vi "Smarthome - server.vi"() -> ()   [LabVIEW 2013]
panel:
  out "URL":string="C:\\Users\\kiat\\Downloads\\asd.mp4"
  in  "WindowsMediaPlayer":refnum<k7>(container)
  out "temperature level 3":bool
  out "Numeric 3":i32
  in  "Slide 3":dbl(slide) scale=16.0..27.0
  out "Ring 6":u16(ring)
  out "check for level 3":bool
  in  "Slide 2":dbl(slide) scale=16.0..27.0
  out "temperature level 2":bool
  out "Numeric 2":i32
  out "Ring 5":u16(ring)
  out "check for level 2":bool
  out "check for level":bool
  in  "Slide":dbl(slide) scale=16.0..27.0
  out "Numeric":i32
  out "temperature level":bool
  out "Ring 4":u16(ring)
  out "Boolean 16":bool
  out "start time 2":string
  out "end time 2":string
  out "Boolean 17":bool
  out "start time 3":string
  out "end time 3":string
  out "end time":string
  out "start time":string
  out "indicator - hour":bool
  out "Bedroom 2":bool
  out "Bedroom 1":bool
  out "Masterroom":bool
  out "For loop count - hour":i32
  in  "stop 3":bool
  out "hour":i32
  out "Ring 3":u16(ring)
  out "Ring 2":u16(ring)
  out "Boolean 15":bool
  in  "stop 2":bool
  out "Boolean 14":bool
  out "Boolean 13":bool
  out "Boolean 12":bool
  out "Boolean 11":bool
  out "Boolean 10":bool
  out "Boolean 9":bool
  out "Boolean 8":bool
  out "Boolean 7":bool
  out "Boolean 6":bool
  out "Boolean 5":bool
  out "Boolean 4":bool
  out "Boolean 3":bool
  out "Boolean 2":bool
  out "Boolean":bool
  out "Boolean 60":bool
  out "Boolean 59":bool
  out "Boolean 58":bool
  out "Boolean 57":bool
  out "Boolean 56":bool
  out "Boolean 55":bool
  out "Boolean 54":bool
  out "Boolean 53":bool
  out "Boolean 52":bool
  out "Boolean 51":bool
  out "Boolean 50":bool
  out "Boolean 49":bool
  out "Boolean 48":bool
  out "Boolean 47":bool
  out "Boolean 46":bool
  out "Boolean 45":bool
  out "Boolean 44":bool
  out "Boolean 43":bool
  out "Boolean 42":bool
  out "Boolean 41":bool
  out "Ring 1":u16(ring)
  in  "stop":bool
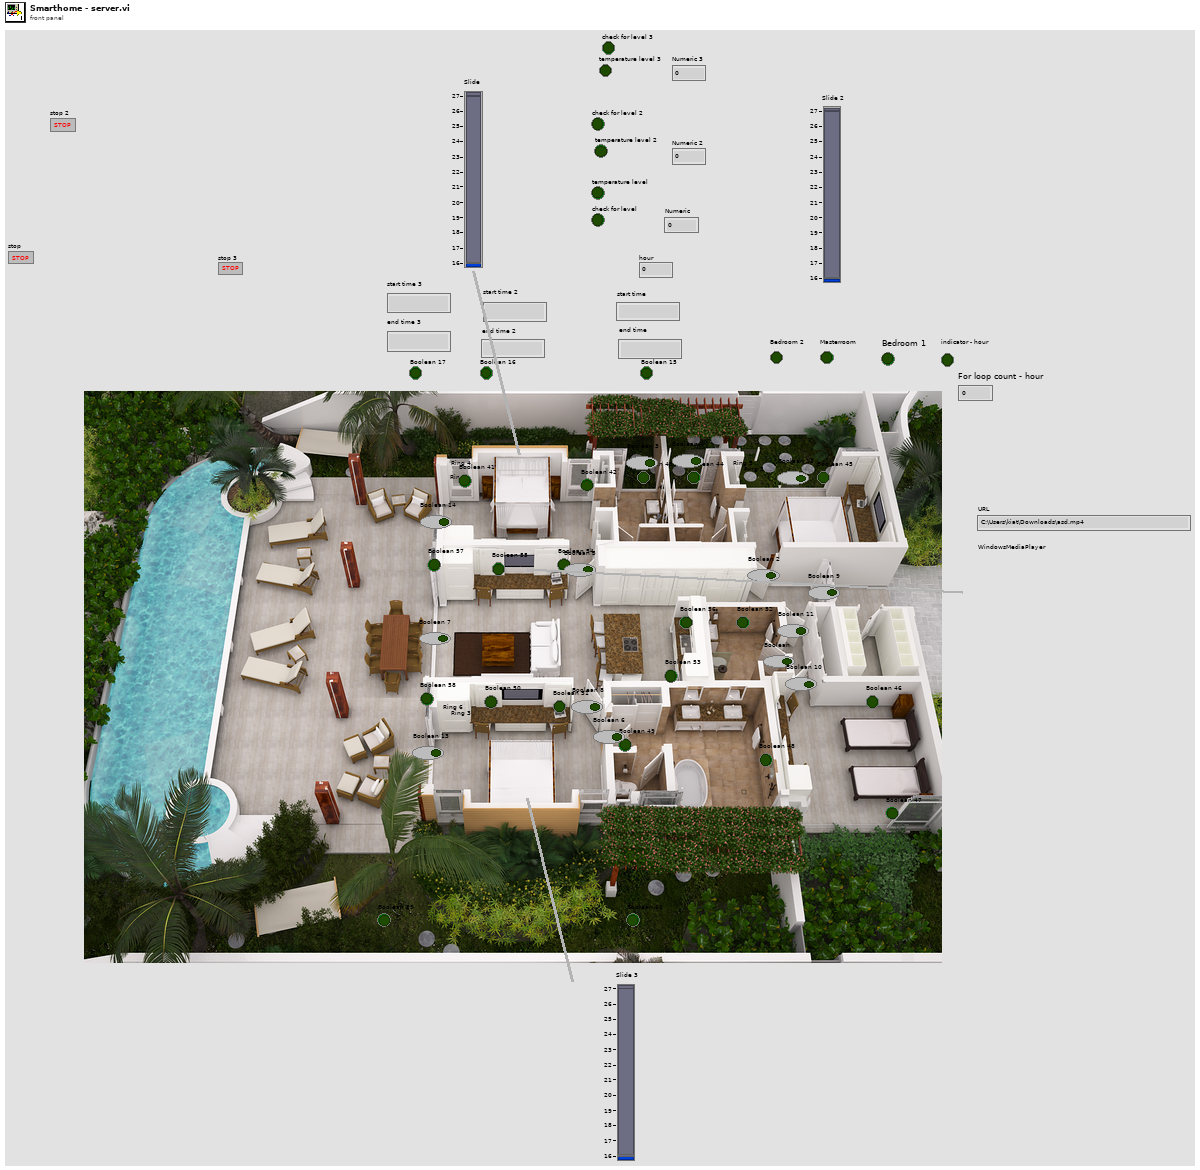
[diagram p1: front panel]
types:
  T1 = cluster{"bytes to read":i32, "Numeric 2":dbl, bool}
  T2 = cluster{"Numeric":dbl, "Numeric 2":dbl, "Numeric 3":dbl, "Numeric 4":dbl, "Numeric 5":dbl, "Numeric 8":dbl, i32, bool}
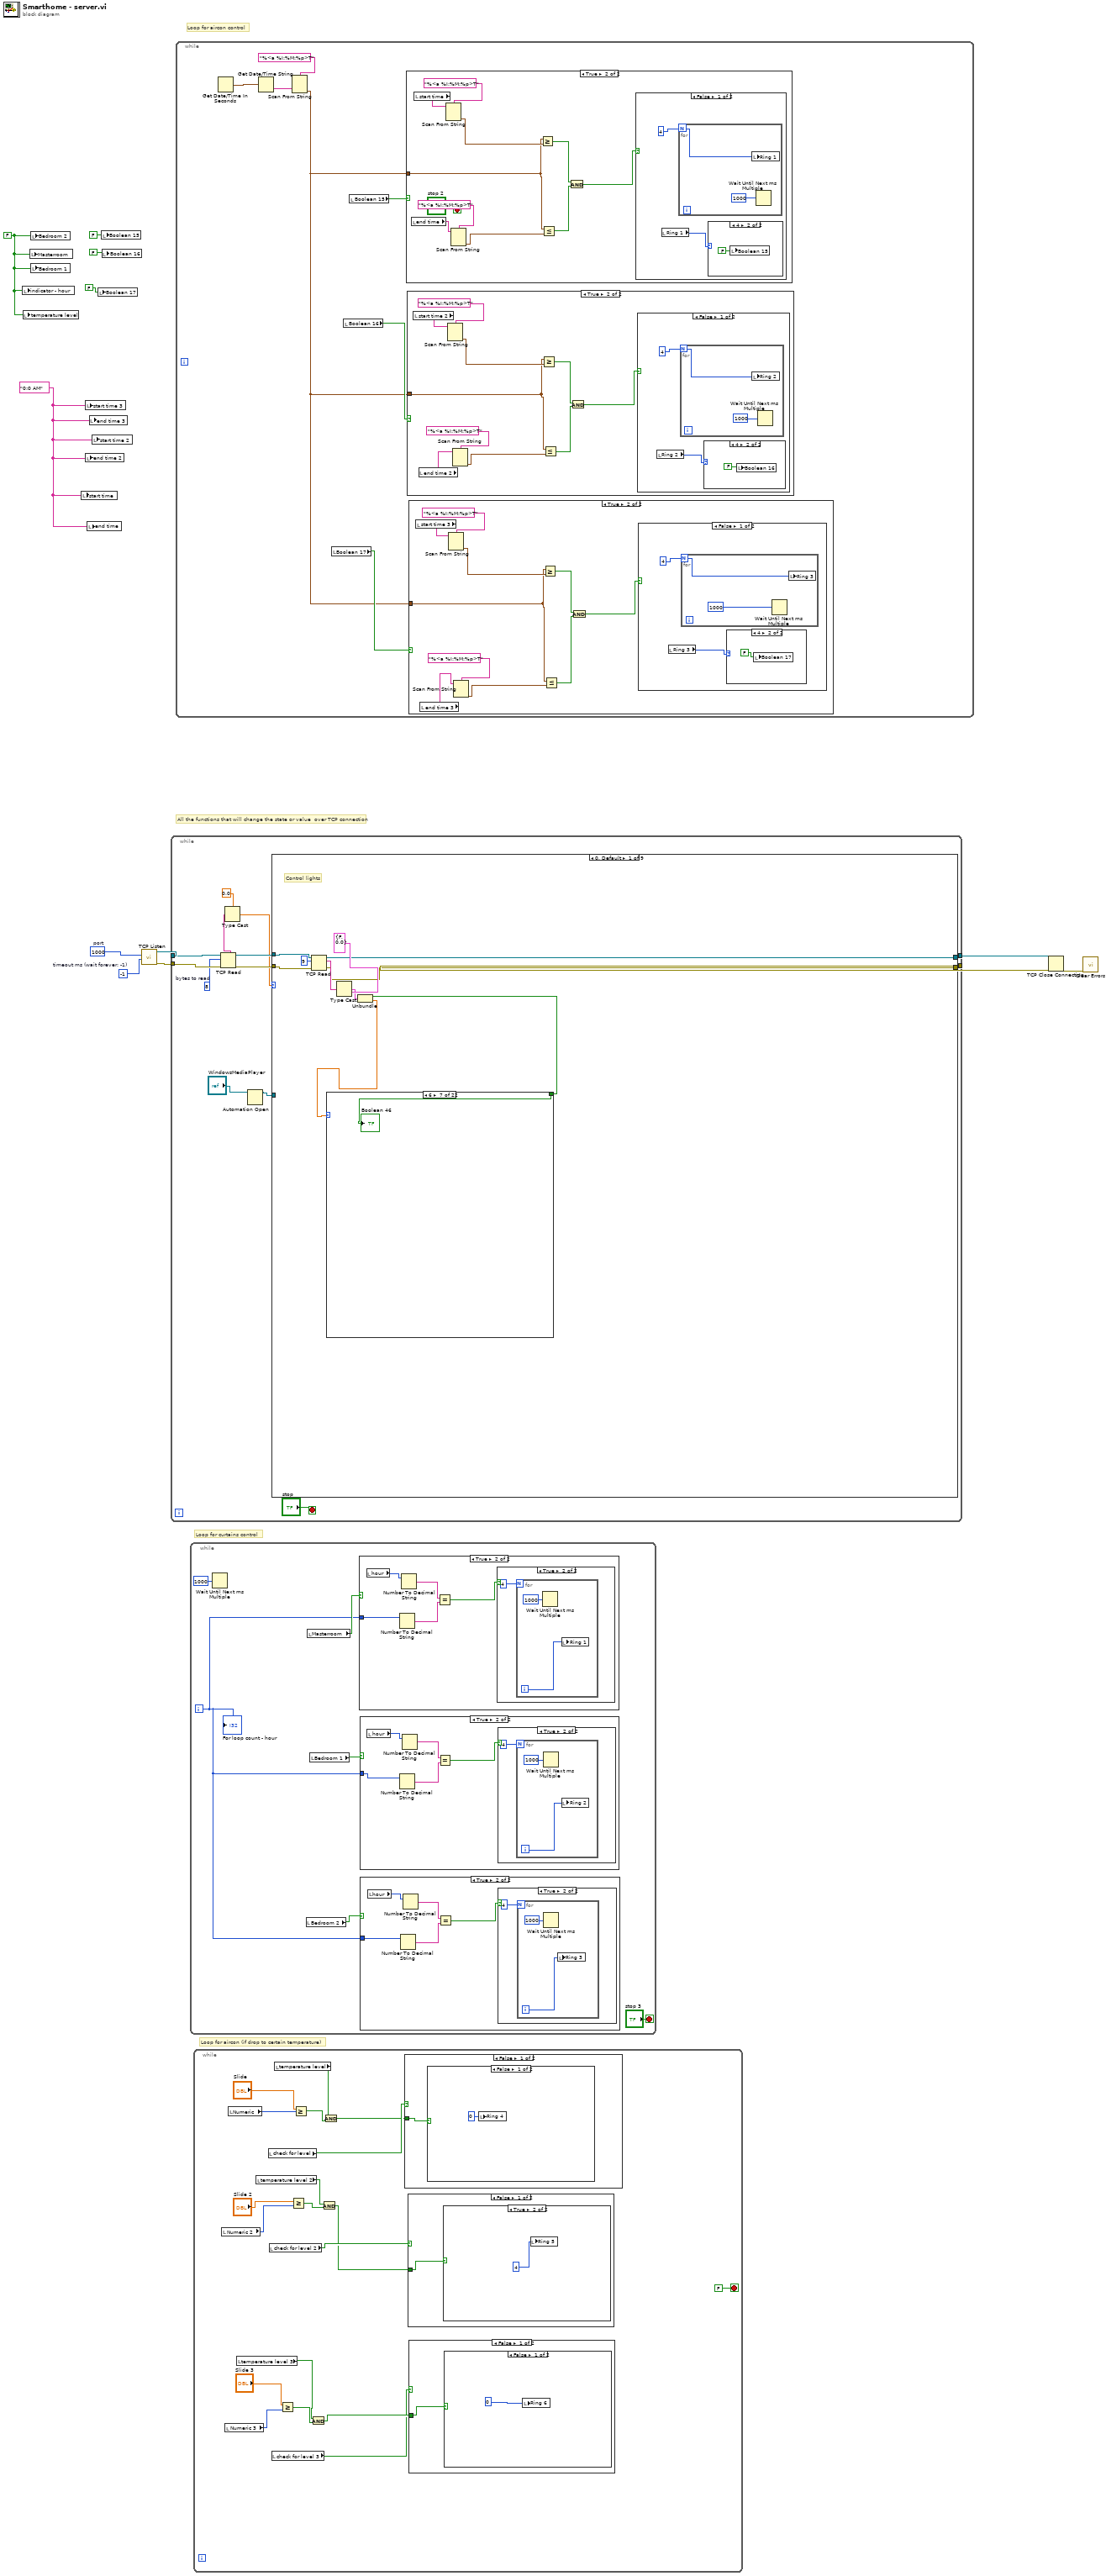
[diagram p0: block diagram]
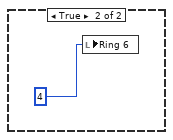
[diagram p2: hidden frame]
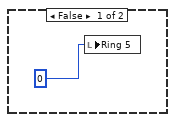
[diagram p4: hidden frame]
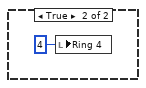
[diagram p6: hidden frame]
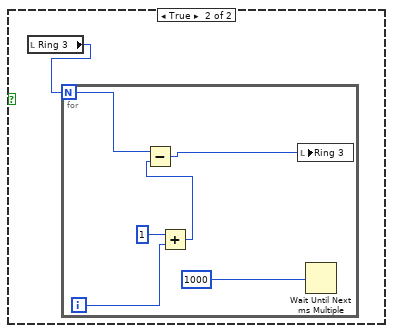
[diagram p16: hidden frame]
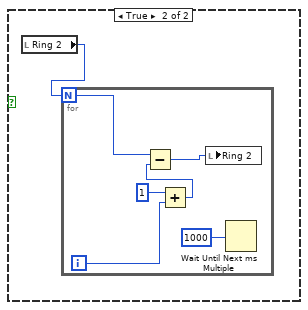
[diagram p19: hidden frame]
diagram:
  w1 = FALSE ("Boolean 15")
  w5 = "0:0 AM"
  w7 = -1  # timeout ms (wait forever: -1)
  w8 = u16 1000  # port
  # "Loop for aircon (if drop to certain temperature)"
  # "Loop for aircon control"
  # "Loop for curtains control"
  # "All the functions that will change the state or value  over TCP connection"
  n1 = local write "indicator - hour"(w1) -> ()
  n2 = local write "temperature level"(w1) -> ()
  n3 = local write "Masterroom"(w1) -> ()
  n4 = local write "Bedroom 2"(w1) -> ()
  n5 = local write "Bedroom 1"(w1) -> ()
  n6 = local write "start time"(w5) -> ()
  n7 = local write "start time 3"(w5) -> ()
  n8 = local write "end time 2"(w5) -> ()
  n9 = local write "end time"(w5) -> ()
  n10 = local write "end time 3"(w5) -> ()
  n11 = local write "start time 2"(w5) -> ()
  n12 = local write "Boolean 17"(FALSE ("Boolean 15")) -> ()
  n13 = local write "Boolean 15"(FALSE ("Boolean 15")) -> ()
  n14 = local write "Boolean 16"(FALSE ("Boolean 15")) -> ()
  n15 = call <vilib>:"TCP Listen.vi"("timeout ms (wait forever: -1)"=w7, "port"=w8) -> ("error out"=w9:errorcluster, "connection ID"=w12:refnum<k5>)  [unwired: 5 in, 3 out]
  n16 = while {
    tunnel: w12 -> [w21]
    tunnel: [w25] -> w11
    tunnel: [w24] -> w10
    tunnel: w9 -> [w22]
    stop <- "stop" stop-if-true
    w18 = 8  # bytes to read
    n17 = TCP Read(connection ID=w21, bytes to read=w18, error in (no error)=w22) -> (connection ID out=w19:refnum<k5>, data out=w17:string, error out=w20:errorcluster)  [unwired: 2 in]
    n18 = Type Cast(type=0.0 ("Numeric"), x=w17) -> (*(type *) &x=w15:dbl)
    n19 = Automation Open(Automation Refnum="WindowsMediaPlayer") -> (Automation Refnum=w13:refnum<k7>)  [unwired: 3 in, 1 out]
    n20 = case shown="0, Default" w15 {
      tunnel: [w30 w65 w77 w122 w209 w235 w317 w334 w359] -> w25
      tunnel: [w31 w64 w76 w121 w210 w236 w318 w335 w360] -> w24
      tunnel: w20 -> [w29 w58 w75 w124 w212 w238 w319 w332 w362]
      tunnel: w19 -> [w28 w57 w74 w123 w213 w237 w320 w333 w361]
      tunnel: w13 -> [_ _ _ _ _ _ _ w330 w355]
      frame 0, Default {
        # "Control lights"
        n21 = TCP Read(connection ID=w28, bytes to read=9, error in (no error)=w29) -> (connection ID out=w30:refnum<k5>, data out=w33:string, error out=w31:errorcluster)  [unwired: 2 in]
        n22 = Type Cast(type=cluster{"Boolean":bool, "Numeric":dbl} {"Boolean"=FALSE, "Numeric"=0.0} ("Cluster"), x=w33) -> (*(type *) &x=w34:cluster{"Boolean":bool, "Numeric":dbl})
        n23 = Unbundle(w34) -> ("Boolean"=w26:bool, "Numeric"=w27:dbl)
        n24 = case shown="6" w27 {
          tunnel: w26 -> [_ w36 w37 w38 w39 w40 w41 w42 w43 w44 w45 w46 w47 w48 _ w49 w50 w51 w52 w53 w54 w55]
          frame 0, Default {
          }
          frame 1 {
            "Boolean 41" <- w36
          }
          frame 2 {
            "Boolean 42" <- w37
          }
          frame 3 {
            "Boolean 43" <- w38
          }
          frame 4 {
            "Boolean 44" <- w39
          }
          frame 5 {
            "Boolean 45" <- w40
          }
          frame 6 {
            "Boolean 46" <- w41
          }
          frame 7 {
            "Boolean 47" <- w42
          }
          frame 8 {
            "Boolean 48" <- w43
          }
          frame 9 {
            "Boolean 49" <- w44
          }
          frame 10 {
            "Boolean 50" <- w45
          }
          frame 11 {
            "Boolean 51" <- w46
          }
          frame 19 {
            "Boolean 52" <- w47
          }
          frame 20 {
            "Boolean 53" <- w48
          }
          frame 21 {
          }
          frame 12 {
            "Boolean 54" <- w49
          }
          frame 13 {
            "Boolean 55" <- w50
          }
          frame 14 {
            "Boolean 56" <- w51
          }
          frame 15 {
            "Boolean 57" <- w52
          }
          frame 16 {
            "Boolean 58" <- w53
          }
          frame 17 {
            "Boolean 59" <- w54
          }
          frame 18 {
            "Boolean 60" <- w55
          }
        }
      }
      frame 1 {
        # "Control curtains"
        n25 = TCP Read(connection ID=w57, bytes to read=16, error in (no error)=w58) -> (connection ID out=w65:refnum<k5>, data out=w62:string, error out=w64:errorcluster)  [unwired: 2 in]
        n26 = Type Cast(type=cluster{"Numeric":dbl, "Numeric 2":dbl} {"Numeric"=0.0, "Numeric 2"=0.0} ("Cluster"), x=w62) -> (*(type *) &x=w61:cluster{"Numeric":dbl, "Numeric 2":dbl})
        n27 = Unbundle(w61) -> ("Numeric"=w56:dbl, "Numeric 2"=w59:dbl)
        n28 = case shown="21" w59 {
          tunnel: w56 -> [_ w66 w67 w68]
          frame 0, Default {
          }
          frame 19 {
            "Ring 1" <- w66
          }
          frame 20 {
            "Ring 2" <- w67
          }
          frame 21 {
            "Ring 3" <- w68
          }
        }
      }
      frame 2 {
        # "Control curtains - set hour"
        n29 = TCP Read(connection ID=w74, bytes to read=13, error in (no error)=w75) -> (connection ID out=w77:refnum<k5>, data out=w80:string, error out=w76:errorcluster)  [unwired: 2 in]
        n30 = Type Cast(type=T1 {"bytes to read"=0, "Numeric 2"=0.0, FALSE} ("Cluster"), x=w80) -> (*(type *) &x=w79:T1)
        n31 = Unbundle(w79) -> ("bytes to read"=w73:i32, "Numeric 2"=w70:dbl, w69:bool)
        "indicator - hour" <- w69
        n32 = case shown="False" w69 {
          tunnel: w70 -> [w82 w86]
          frame False {
            n33 = case shown="24" w82 {
              frame 0, Default {
              }
              frame 22 {
                n34 = local read "indicator - hour"() -> (→"Masterroom":bool)
              }
              frame 23 {
                n35 = local read "indicator - hour"() -> (→"Bedroom 1":bool)
              }
              frame 24 {
                n36 = local read "indicator - hour"() -> (→"Bedroom 2":bool)
              }
            }
          }
          frame True {
            n37 = case shown="22" w86 {
              frame 0, Default {
              }
              frame 22 {
                n38 = local read "Ring 1"() -> (w88:u16)
                n39 = local read "indicator - hour"() -> (w87:bool)
                n40 = for {
                  N: w88 -> [_]
                  tunnel: w88 -> [w94]
                  i -> [w91]
                  n41 = Add(x=1, y=w91) -> (x+y=w89:i32)
                  n42 = Subtract(x=w94, y=w89) -> (x-y=w93:i32)
                  n43 = local write "Ring 1"(w93) -> ()
                  n44 = Wait Until Next ms Multiple(millisecond multiple=u32 1000) -> ()  [unwired: 1 out]
                }
                n45 = local write "Masterroom"(w87) -> ()
              }
              frame 23 {
                n46 = local read "Ring 2"() -> (w96:u16)
                n47 = local read "indicator - hour"() -> (w95:bool)
                n48 = for {
                  N: w96 -> [_]
                  tunnel: w96 -> [w102]
                  i -> [w100]
                  n49 = Add(x=1, y=w100) -> (x+y=w98:i32)
                  n50 = Subtract(x=w102, y=w98) -> (x-y=w97:i32)
                  n51 = local write "Ring 2"(w97) -> ()
                  n52 = Wait Until Next ms Multiple(millisecond multiple=u32 1000) -> ()  [unwired: 1 out]
                }
                n53 = local write "Bedroom 1"(w95) -> ()
              }
              frame 24 {
                n54 = local read "indicator - hour"() -> (w103:bool)
                n55 = local read "Ring 3"() -> (w104:u16)
                n56 = for {
                  N: w104 -> [_]
                  tunnel: w104 -> [w110]
                  i -> [w108]
                  n57 = Add(x=1, y=w108) -> (x+y=w106:i32)
                  n58 = Subtract(x=w110, y=w106) -> (x-y=w105:i32)
                  n59 = Wait Until Next ms Multiple(millisecond multiple=u32 1000) -> ()  [unwired: 1 out]
                  n60 = local write "Ring 3"(w105) -> ()
                }
                n61 = local write "Bedroom 2"(w103) -> ()
              }
            }
          }
        }
        n62 = local read "For loop count - hour"() -> (w71:i32)
        n63 = Add(x=w73, y=w71) -> (x+y=→"hour":i32)
      }
      frame 3 {
        # "Control curtains - in specific time"
        n64 = TCP Read(connection ID=w123, bytes to read=53, error in (no error)=w124) -> (connection ID out=w122:refnum<k5>, data out=w125:string, error out=w121:errorcluster)  [unwired: 2 in]
        n65 = Type Cast(type=T2 {"Numeric"=0.0, "Numeric 2"=0.0, "Numeric 3"=0.0, "Numeric 4"=0.0, "Numeric 5"=0.0, "Numeric 8"=0.0, 0, TRUE} ("Cluster"), x=w125) -> (*(type *) &x=w119:T2)
        n66 = Unbundle(w119) -> ("Numeric"=w117:dbl, "Numeric 2"=w118:dbl, "Numeric 3"=w114:dbl, "Numeric 4"=w113:dbl, "Numeric 5"=w116:dbl, "Numeric 8"=w112:dbl, w111:i32, w115:bool)
        n67 = case shown="1" w111 {
          tunnel: w115 -> [_ w147 w161 w183]
          tunnel: w118 -> [_ w149 w158 w184]
          tunnel: w117 -> [_ w148 w154 w188]
          tunnel: w116 -> [_ w141 w155 w187]
          tunnel: w114 -> [_ w137 w156 w186]
          tunnel: w113 -> [_ w136 w157 w185]
          tunnel: w112 -> [_ w135 w162 w182]
          frame 0, Default {
          }
          frame 1 {
            n68 = To Long Integer(number=w136) -> (32bit integer=w129:i32)
            n69 = To Long Integer(number=w137) -> (32bit integer=w130:i32)
            n70 = To Long Integer(number=w135) -> (32bit integer=w134:i32)
            n71 = case shown="0, Default" w134 {
              tunnel: [" AM" " PM"] -> w128
              frame 0, Default {
              }
              frame 1 {
              }
            }
            n72 = Number To Decimal String(number=w129) -> (decimal integer string=w132:string)  [unwired: 1 in]
            n73 = Number To Decimal String(number=w130) -> (decimal integer string=w131:string)  [unwired: 1 in]
            n74 = To Long Integer(number=w149) -> (32bit integer=w145:i32)
            n75 = To Long Integer(number=w148) -> (32bit integer=w146:i32)
            n76 = Number To Decimal String(number=w145) -> (decimal integer string=w143:string)  [unwired: 1 in]
            n77 = Concatenate Strings(w131, ":" ("string"), w132, w128) -> (→"end time":string)
            n78 = Number To Decimal String(number=w146) -> (decimal integer string=w144:string)  [unwired: 1 in]
            n79 = To Long Integer(number=w141) -> (32bit integer=w140:i32)
            n80 = case shown="1" w140 {
              tunnel: [" AM" " PM"] -> w139
              frame 0, Default {
              }
              frame 1 {
              }
            }
            n81 = Concatenate Strings(w144, ":" ("string"), w143, w139) -> (→"start time":string)
            "Boolean 15" <- w147
          }
          frame 2 {
            n82 = To Long Integer(number=w157) -> (32bit integer=w164:i32)
            n83 = To Long Integer(number=w156) -> (32bit integer=w165:i32)
            n84 = To Long Integer(number=w162) -> (32bit integer=w160:i32)
            n85 = case shown="1" w160 {
              tunnel: [" AM" " PM"] -> w159
              frame 0, Default {
              }
              frame 1 {
              }
            }
            n86 = Number To Decimal String(number=w164) -> (decimal integer string=w167:string)  [unwired: 1 in]
            n87 = Number To Decimal String(number=w165) -> (decimal integer string=w166:string)  [unwired: 1 in]
            n88 = To Long Integer(number=w158) -> (32bit integer=w175:i32)
            n89 = To Long Integer(number=w154) -> (32bit integer=w176:i32)
            n90 = Number To Decimal String(number=w175) -> (decimal integer string=w173:string)  [unwired: 1 in]
            n91 = Concatenate Strings(w166, ":" ("string"), w167, w159) -> (→"end time 2":string)
            n92 = Number To Decimal String(number=w176) -> (decimal integer string=w174:string)  [unwired: 1 in]
            n93 = To Long Integer(number=w155) -> (32bit integer=w171:i32)
            n94 = case shown="1" w171 {
              tunnel: [" AM" " PM"] -> w170
              frame 0, Default {
              }
              frame 1 {
              }
            }
            n95 = Concatenate Strings(w174, ":" ("string"), w173, w170) -> (→"start time 2":string)
            "Boolean 16" <- w161
          }
          frame 3 {
            n96 = To Long Integer(number=w185) -> (32bit integer=w190:i32)
            n97 = To Long Integer(number=w186) -> (32bit integer=w191:i32)
            n98 = To Long Integer(number=w182) -> (32bit integer=w195:i32)
            n99 = case shown="0, Default" w195 {
              tunnel: [" AM" " PM"] -> w189
              frame 0, Default {
              }
              frame 1 {
              }
            }
            n100 = Number To Decimal String(number=w190) -> (decimal integer string=w193:string)  [unwired: 1 in]
            n101 = Number To Decimal String(number=w191) -> (decimal integer string=w192:string)  [unwired: 1 in]
            n102 = To Long Integer(number=w184) -> (32bit integer=w202:i32)
            n103 = To Long Integer(number=w188) -> (32bit integer=w203:i32)
            n104 = Number To Decimal String(number=w202) -> (decimal integer string=w200:string)  [unwired: 1 in]
            n105 = Concatenate Strings(w192, ":" ("string"), w193, w189) -> (→"end time 3":string)
            n106 = Number To Decimal String(number=w203) -> (decimal integer string=w201:string)  [unwired: 1 in]
            n107 = To Long Integer(number=w187) -> (32bit integer=w198:i32)
            n108 = case shown="1" w198 {
              tunnel: [" AM" " PM"] -> w197
              frame 0, Default {
              }
              frame 1 {
              }
            }
            n109 = Concatenate Strings(w201, ":" ("string"), w200, w197) -> (→"start time 3":string)
            "Boolean 17" <- w183
          }
        }
      }
      frame 4 {
        # "Control door"
        n110 = TCP Read(connection ID=w213, bytes to read=9, error in (no error)=w212) -> (connection ID out=w209:refnum<k5>, data out=w216:string, error out=w210:errorcluster)  [unwired: 2 in]
        n111 = Type Cast(type=cluster{bool, "Numeric 2":dbl} {TRUE, "Numeric 2"=0.0} ("Cluster"), x=w216) -> (*(type *) &x=w215:cluster{bool, "Numeric 2":dbl})
        n112 = Unbundle(w215) -> (w208:bool, "Numeric 2"=w214:dbl)
        n113 = case shown="5" w214 {
          tunnel: w208 -> [_ w218 w219 w220 w221 w222 w223 w224 w225 w226 w227 w228 w229 w230 w231]
          frame 0, Default {
          }
          frame 1 {
            "Boolean 5" <- w218
          }
          frame 2 {
            "Boolean 14" <- w219
          }
          frame 3 {
            "Boolean 8" <- w220
          }
          frame 4 {
            "Boolean 13" <- w221
          }
          frame 5 {
            "Boolean 2" <- w222
          }
          frame 6 {
            "Boolean 12" <- w223
          }
          frame 7 {
            "Boolean 10" <- w224
          }
          frame 8 {
            "Boolean 3" <- w225
          }
          frame 9 {
            "Boolean 6" <- w226
          }
          frame 10 {
            "Boolean 4" <- w227
          }
          frame 11 {
            "Boolean" <- w228
          }
          frame 12 {
            "Boolean 9" <- w229
          }
          frame 13 {
            "Boolean 11" <- w230
          }
          frame 14 {
            "Boolean 7" <- w231
          }
        }
      }
      frame 5 {
        # "Control air con"
        n114 = TCP Read(connection ID=w237, bytes to read=17, error in (no error)=w238) -> (connection ID out=w235:refnum<k5>, data out=w242:string, error out=w236:errorcluster)  [unwired: 2 in]
        n115 = Type Cast(type=cluster{bool, "Numeric 2":dbl, "Numeric 3":dbl} {TRUE, "Numeric 2"=0.0, "Numeric 3"=0.0} ("Cluster"), x=w242) -> (*(type *) &x=w241:cluster{bool, "Numeric 2":dbl, "Numeric 3":dbl})
        n116 = Unbundle(w241) -> (w232:bool, "Numeric 2"=w233:dbl, "Numeric 3"=w234:dbl)
        n117 = case shown="True" w232 {
          tunnel: w234 -> [w243 w252]
          tunnel: w233 -> [_ w251]
          tunnel: w232 -> [_ w250]
          frame False {
            n118 = case shown="2" w243 {
              frame 0, Default {
              }
              frame 1 {
                n119 = local write "check for level"(FALSE ("check for level 2")) -> ()
                n120 = local write "Ring 4"(u16 0 ("Ring 4")) -> ()
              }
              frame 2 {
                n121 = local write "check for level 2"(FALSE ("check for level")) -> ()
                n122 = local write "Ring 5"(u16 0 ("Ring 5")) -> ()
              }
              frame 3 {
                n123 = local write "check for level 3"(FALSE ("check for level")) -> ()
                n124 = local write "Ring 6"(u16 0 ("Ring 5")) -> ()
              }
            }
          }
          frame True {
            n125 = case shown="2" w252 {
              tunnel: w251 -> [_ w254 w273 w293]
              tunnel: w250 -> [_ w253 w274 w294]
              frame 0, Default {
              }
              frame 1 {
                w258 = 16.0 ("y")
                w266 = 21.0 ("y")
                w267 = 24.0 ("y")
                n126 = local write "Slide"(w254) -> ()
                n127 = Less Or Equal?(x=w254, y=27.0) -> (x <= y?=w261:bool)
                n128 = Less Or Equal?(x=w254, y=w267) -> (x <= y?=w260:bool)
                n129 = Greater?(x=w254, y=w266) -> (0:w259:bool)
                n130 = Greater?(x=w254, y=w258) -> (0:w256:bool)
                n131 = Less Or Equal?(x=w254, y=w266) -> (x <= y?=w257:bool)
                n132 = Greater?(x=w254, y=w267) -> (0:w262:bool)
                n133 = Less Or Equal?(x=w254, y=w258) -> (x <= y?=w255:bool)
                n134 = And(x=w261, y=w262) -> (x .and. y?=w263:bool)
                n135 = And(x=w260, y=w259) -> (x .and. y?=w265:bool)
                n136 = And(x=w257, y=w256) -> (x .and. y?=w264:bool)
                n137 = case shown="True" w263 {
                  frame False {
                  }
                  frame True {
                    "Ring 4" <- u16 1 ("Ring 4")
                  }
                }
                n138 = case shown="True" w265 {
                  frame False {
                  }
                  frame True {
                    n139 = local write "Ring 4"(u16 2 ("Ring 4")) -> ()
                  }
                }
                n140 = case shown="True" w264 {
                  frame False {
                  }
                  frame True {
                    n141 = local write "Ring 4"(u16 3 ("Ring 4")) -> ()
                  }
                }
                n142 = case shown="True" w255 {
                  frame False {
                  }
                  frame True {
                    n143 = local write "Ring 4"(u16 4 ("Ring 4")) -> ()
                  }
                }
                "check for level" <- w253
              }
              frame 2 {
                w278 = 16.0 ("y")
                w286 = 21.0 ("y")
                w287 = 24.0 ("y")
                n144 = local write "Slide 2"(w273) -> ()
                n145 = Less Or Equal?(x=w273, y=27.0) -> (x <= y?=w281:bool)
                n146 = Less Or Equal?(x=w273, y=w287) -> (x <= y?=w280:bool)
                n147 = Greater?(x=w273, y=w286) -> (0:w279:bool)
                n148 = Greater?(x=w273, y=w278) -> (0:w276:bool)
                n149 = Less Or Equal?(x=w273, y=w286) -> (x <= y?=w277:bool)
                n150 = Greater?(x=w273, y=w287) -> (0:w282:bool)
                n151 = Less Or Equal?(x=w273, y=w278) -> (x <= y?=w275:bool)
                n152 = And(x=w281, y=w282) -> (x .and. y?=w283:bool)
                n153 = And(x=w280, y=w279) -> (x .and. y?=w285:bool)
                n154 = And(x=w277, y=w276) -> (x .and. y?=w284:bool)
                n155 = case shown="True" w283 {
                  frame False {
                  }
                  frame True {
                    "Ring 5" <- u16 1 ("Ring 4")
                  }
                }
                n156 = case shown="True" w285 {
                  frame False {
                  }
                  frame True {
                    n157 = local write "Ring 5"(u16 2 ("Ring 4")) -> ()
                  }
                }
                n158 = case shown="True" w284 {
                  frame False {
                  }
                  frame True {
                    n159 = local write "Ring 5"(u16 3 ("Ring 4")) -> ()
                  }
                }
                n160 = case shown="True" w275 {
                  frame False {
                  }
                  frame True {
                    n161 = local write "Ring 5"(u16 4 ("Ring 4")) -> ()
                  }
                }
                "check for level 2" <- w274
              }
              frame 3 {
                w298 = 16.0 ("y")
                w306 = 21.0 ("y")
                w307 = 24.0 ("y")
                n162 = local write "Slide 3"(w293) -> ()
                n163 = Less Or Equal?(x=w293, y=27.0) -> (x <= y?=w301:bool)
                n164 = Less Or Equal?(x=w293, y=w307) -> (x <= y?=w300:bool)
                n165 = Greater?(x=w293, y=w306) -> (0:w299:bool)
                n166 = Greater?(x=w293, y=w298) -> (0:w296:bool)
                n167 = Less Or Equal?(x=w293, y=w306) -> (x <= y?=w297:bool)
                n168 = Greater?(x=w293, y=w307) -> (0:w302:bool)
                n169 = Less Or Equal?(x=w293, y=w298) -> (x <= y?=w295:bool)
                n170 = And(x=w301, y=w302) -> (x .and. y?=w303:bool)
                n171 = And(x=w300, y=w299) -> (x .and. y?=w305:bool)
                n172 = And(x=w297, y=w296) -> (x .and. y?=w304:bool)
                n173 = case shown="True" w303 {
                  frame False {
                  }
                  frame True {
                    "Ring 6" <- u16 1 ("Ring 4")
                  }
                }
                n174 = case shown="True" w305 {
                  frame False {
                  }
                  frame True {
                    n175 = local write "Ring 6"(u16 2 ("Ring 4")) -> ()
                  }
                }
                n176 = case shown="True" w304 {
                  frame False {
                  }
                  frame True {
                    n177 = local write "Ring 6"(u16 3 ("Ring 4")) -> ()
                  }
                }
                n178 = case shown="True" w295 {
                  frame False {
                  }
                  frame True {
                    n179 = local write "Ring 6"(u16 4 ("Ring 4")) -> ()
                  }
                }
                "check for level 3" <- w294
              }
            }
          }
        }
      }
      frame 6 {
        # "Control air con - if drop to certain temperature"
        n180 = TCP Read(connection ID=w320, bytes to read=13, error in (no error)=w319) -> (connection ID out=w317:refnum<k5>, data out=w322:string, error out=w318:errorcluster)  [unwired: 2 in]
        n181 = Type Cast(type=cluster{bool, i32, "Numeric 2":dbl} {TRUE, 0, "Numeric 2"=0.0} ("Cluster"), x=w322) -> (*(type *) &x=w321:cluster{bool, i32, "Numeric 2":dbl})
        n182 = Unbundle(w321) -> (w314:bool, w313:i32, "Numeric 2"=w315:dbl)
        n183 = case shown="3" w315 {
          tunnel: w314 -> [_ w325 w326 w328]
          tunnel: w313 -> [_ w324 w327 w329]
          frame 0, Default {
          }
          frame 1 {
            "temperature level" <- w325
            "Numeric" <- w324
          }
          frame 2 {
            "temperature level 2" <- w326
            "Numeric 2" <- w327
          }
          frame 3 {
            "temperature level 3" <- w328
            "Numeric 3" <- w329
          }
        }
      }
      frame 7 {
        # "Control TV -action"
        n184 = TCP Read(connection ID=w333, bytes to read=8, error in (no error)=w332) -> (connection ID out=w334:refnum<k5>, data out=w337:string, error out=w335:errorcluster)  [unwired: 2 in]
        n185 = Type Cast(type=cluster{"Numeric 2":dbl} {"Numeric 2"=0.0} ("Cluster"), x=w337) -> (*(type *) &x=w338:cluster{"Numeric 2":dbl})
        n186 = Unbundle(w338) -> ("Numeric 2"=w331:dbl)
        n187 = case shown="6" w331 {
          tunnel: w330 -> [_ w340 w343 w346 w349 w352]
          frame 0, Default {
          }
          frame 2 {
            n188 = property class="IWMPPlayer4"(reference=w340) -> ("controls"=w341:refnum<k7>)  [unwired: 1 in, 2 out]
            n189 = invoke class="IWMPControls" method="play"(reference=w341) -> (reference out=w342:refnum<k7>)  [unwired: 2 in, 2 out]
            n190 = Close Reference(reference=w342) -> ()  [unwired: 1 in, 1 out]
          }
          frame 3 {
            n191 = property class="IWMPPlayer4"(reference=w343) -> ("controls"=w345:refnum<k7>)  [unwired: 1 in, 2 out]
            n192 = invoke class="IWMPControls" method="pause"(reference=w345) -> (reference out=w344:refnum<k7>)  [unwired: 2 in, 2 out]
            n193 = Close Reference(reference=w344) -> ()  [unwired: 1 in, 1 out]
          }
          frame 4 {
            n194 = property class="IWMPPlayer4"(reference=w346) -> ("controls"=w347:refnum<k7>)  [unwired: 1 in, 2 out]
            n195 = invoke class="IWMPControls" method="stop"(reference=w347) -> (reference out=w348:refnum<k7>)  [unwired: 2 in, 2 out]
            n196 = Close Reference(reference=w348) -> ()  [unwired: 1 in, 1 out]
          }
          frame 5 {
            n197 = property class="IWMPPlayer4"(reference=w349) -> ("controls"=w350:refnum<k7>)  [unwired: 1 in, 2 out]
            n198 = invoke class="IWMPControls" method="fastReverse"(reference=w350) -> (reference out=w351:refnum<k7>)  [unwired: 2 in, 2 out]
            n199 = Close Reference(reference=w351) -> ()  [unwired: 1 in, 1 out]
          }
          frame 6 {
            n200 = property class="IWMPPlayer4"(reference=w352) -> ("controls"=w354:refnum<k7>)  [unwired: 1 in, 2 out]
            n201 = invoke class="IWMPControls" method="fastForward"(reference=w354) -> (reference out=w353:refnum<k7>)  [unwired: 2 in, 2 out]
            n202 = Close Reference(reference=w353) -> ()  [unwired: 1 in, 1 out]
          }
        }
      }
      frame 8 {
        # "Control TV"
        n203 = TCP Read(connection ID=w361, bytes to read=16, error in (no error)=w362) -> (connection ID out=w359:refnum<k5>, data out=w364:string, error out=w360:errorcluster)  [unwired: 2 in]
        n204 = Type Cast(type=cluster{"Numeric 2":dbl, "Numeric 3":dbl} {"Numeric 2"=0.0, "Numeric 3"=0.0} ("Cluster"), x=w364) -> (*(type *) &x=w365:cluster{"Numeric 2":dbl, "Numeric 3":dbl})
        n205 = Unbundle(w365) -> ("Numeric 2"=w356:dbl, "Numeric 3"=w357:dbl)
        n206 = case shown="1" w357 {
          tunnel: w356 -> [_ w371 w375]
          tunnel: w355 -> [_ w367 w376]
          frame 0, Default {
          }
          frame 1 {
            n207 = case shown="0, Default" w371 {
              frame 0, Default {
                "URL" <- "C:\\Users\\kiat\\Downloads\\asd.mp4" ("URL")
              }
              frame 1 {
                n208 = local write "URL"("C:\\Users\\kiat\\Downloads\\videoplayback.mp4" ("URL")) -> ()
              }
              frame 2 {
                n209 = local write "URL"("C:\\Users\\kiat\\Downloads\\wiggle.mp4" ("URL")) -> ()
              }
            }
            n210 = local read "URL"() -> (w366:string)
            n211 = property class="IWMPPlayer4"(reference=w367, "URL"=w366) -> (reference out=w370:refnum<k7>)  [unwired: 1 in, 1 out]
            n212 = property class="IWMPPlayer4"(reference=w370) -> ("controls"=w369:refnum<k7>)  [unwired: 1 in, 2 out]
            n213 = invoke class="IWMPControls" method="play"(reference=w369) -> (reference out=w368:refnum<k7>)  [unwired: 2 in, 2 out]
            n214 = Close Reference(reference=w368) -> ()  [unwired: 1 in, 1 out]
          }
          frame 2 {
            n215 = property class="IWMPPlayer4"(reference=w376) -> ("settings"=w378:refnum<k7>)  [unwired: 1 in, 2 out]
            n216 = property class="IWMPSettings"(reference=w378, "volume"=w375) -> (reference out=w377:refnum<k7>)  [unwired: 1 in, 1 out]
            n217 = Close Reference(reference=w377) -> ()  [unwired: 1 in, 1 out]
          }
        }
      }
    }
  }
  n218 = while {
    stop <- "stop 2" stop-if-true
    n219 = Get Date/Time In Seconds() -> (seconds since 1Jan1904=w384:timestamp)
    n220 = Get Date/Time String(seconds (now)=w384) -> (time string=w383:string)  [unwired: 2 in, 1 out]
    n221 = Scan From String(format string="%<a %I:%M:%p>T" ("input string"), input string=w383) -> (output 1=w380:timestamp)  [unwired: 3 in, 3 out]
    n222 = local read "Boolean 17"() -> (w381:bool)
    n223 = local read "Boolean 16"() -> (w382:bool)
    n224 = local read "Boolean 15"() -> (w385:bool)
    n225 = case shown="True" w385 {
      tunnel: w380 -> [_ w436]
      frame False {
      }
      frame True {
        n226 = local read "end time"() -> (w438:string)
        n227 = local read "start time"() -> (w440:string)
        n228 = Scan From String(format string="%<a %I:%M:%p>T" ("input string"), input string=w440) -> (output 1=w439:timestamp)  [unwired: 3 in, 3 out]
        n229 = Scan From String(format string="%<a %I:%M:%p>T" ("input string"), input string=w438) -> (output 1=w437:timestamp)  [unwired: 3 in, 3 out]
        n230 = Greater Or Equal?(x=w436, y=w439) -> (x >= y?=w434:bool)
        n231 = Less Or Equal?(x=w436, y=w437) -> (x <= y?=w435:bool)
        n232 = And(x=w434, y=w435) -> (x .and. y?=w433:bool)
        n233 = case shown="False" w433 {
          frame False {
            n234 = local read "Ring 1"() -> (w441:u16)
            n235 = for {
              N: 4 -> [w444]
              n236 = local write "Ring 1"(w444) -> ()
              n237 = Wait Until Next ms Multiple(millisecond multiple=u32 1000) -> ()  [unwired: 1 out]
            }
            n238 = case shown="4" w441 {
              frame 0, Default {
              }
              frame 4 {
                n239 = local write "Boolean 15"(FALSE ("Boolean 15")) -> ()
              }
            }
          }
          frame True {
            n240 = local read "Ring 1"() -> (w446:u16)
            n241 = for {
              N: w446 -> [w447]
              i -> [w448]
              n242 = Add(x=1, y=w448) -> (x+y=w451:i32)
              n243 = Subtract(x=w447, y=w451) -> (x-y=w449:i32)
              n244 = local write "Ring 1"(w449) -> ()
              n245 = Wait Until Next ms Multiple(millisecond multiple=u32 1000) -> ()  [unwired: 1 out]
            }
          }
        }
      }
    }
    n246 = case shown="True" w382 {
      tunnel: w380 -> [_ w416]
      frame False {
      }
      frame True {
        n247 = local read "start time 2"() -> (w412:string)
        n248 = local read "end time 2"() -> (w411:string)
        n249 = Scan From String(format string="%<a %I:%M:%p>T" ("input string"), input string=w412) -> (output 1=w418:timestamp)  [unwired: 3 in, 3 out]
        n250 = Scan From String(format string="%<a %I:%M:%p>T" ("input string"), input string=w411) -> (output 1=w417:timestamp)  [unwired: 3 in, 3 out]
        n251 = Greater Or Equal?(x=w416, y=w418) -> (x >= y?=w414:bool)
        n252 = Less Or Equal?(x=w416, y=w417) -> (x <= y?=w415:bool)
        n253 = And(x=w414, y=w415) -> (x .and. y?=w413:bool)
        n254 = case shown="False" w413 {
          frame False {
            n255 = local read "Ring 2"() -> (w419:u16)
            n256 = for {
              N: 4 -> [w422]
              n257 = local write "Ring 2"(w422) -> ()
              n258 = Wait Until Next ms Multiple(millisecond multiple=u32 1000) -> ()  [unwired: 1 out]
            }
            n259 = case shown="4" w419 {
              frame 0, Default {
              }
              frame 4 {
                n260 = local write "Boolean 16"(FALSE ("Boolean 15")) -> ()
              }
            }
          }
          frame True {
            n261 = local read "Ring 2"() -> (w424:u16)
            n262 = for {
              N: w424 -> [w426]
              i -> [w427]
              n263 = Add(x=1, y=w427) -> (x+y=w429:i32)
              n264 = Subtract(x=w426, y=w429) -> (x-y=w425:i32)
              n265 = local write "Ring 2"(w425) -> ()
              n266 = Wait Until Next ms Multiple(millisecond multiple=u32 1000) -> ()  [unwired: 1 out]
            }
          }
        }
      }
    }
    n267 = case shown="True" w381 {
      tunnel: w380 -> [_ w394]
      frame False {
      }
      frame True {
        n268 = local read "start time 3"() -> (w390:string)
        n269 = local read "end time 3"() -> (w389:string)
        n270 = Scan From String(format string="%<a %I:%M:%p>T" ("input string"), input string=w390) -> (output 1=w396:timestamp)  [unwired: 3 in, 3 out]
        n271 = Scan From String(format string="%<a %I:%M:%p>T" ("input string"), input string=w389) -> (output 1=w395:timestamp)  [unwired: 3 in, 3 out]
        n272 = Greater Or Equal?(x=w394, y=w396) -> (x >= y?=w392:bool)
        n273 = Less Or Equal?(x=w394, y=w395) -> (x <= y?=w393:bool)
        n274 = And(x=w392, y=w393) -> (x .and. y?=w391:bool)
        n275 = case shown="False" w391 {
          frame False {
            n276 = local read "Ring 3"() -> (w397:u16)
            n277 = for {
              N: 4 -> [w400]
              n278 = Wait Until Next ms Multiple(millisecond multiple=u32 1000) -> ()  [unwired: 1 out]
              n279 = local write "Ring 3"(w400) -> ()
            }
            n280 = case shown="4" w397 {
              frame 0, Default {
              }
              frame 4 {
                n281 = local write "Boolean 17"(FALSE ("Boolean 15")) -> ()
              }
            }
          }
          frame True {
            n282 = local read "Ring 3"() -> (w402:u16)
            n283 = for {
              N: w402 -> [w404]
              i -> [w405]
              n284 = Add(x=1, y=w405) -> (x+y=w407:i32)
              n285 = Subtract(x=w404, y=w407) -> (x-y=w403:i32)
              n286 = local write "Ring 3"(w403) -> ()
              n287 = Wait Until Next ms Multiple(millisecond multiple=u32 1000) -> ()  [unwired: 1 out]
            }
          }
        }
      }
    }
  }
  n288 = while {
    i -> [w453]
    stop <- "stop 3" stop-if-true
    n289 = Wait Until Next ms Multiple(millisecond multiple=u32 1000) -> ()  [unwired: 1 out]
    n290 = local read "Bedroom 2"() -> (w454:bool)
    n291 = local read "Masterroom"() -> (w456:bool)
    n292 = local read "Bedroom 1"() -> (w455:bool)
    n293 = case shown="True" w456 {
      tunnel: w453 -> [_ w479]
      frame False {
      }
      frame True {
        n294 = local read "hour"() -> (w476:i32)
        n295 = Number To Decimal String(number=w479) -> (decimal integer string=w478:string)  [unwired: 1 in]
        n296 = Number To Decimal String(number=w476) -> (decimal integer string=w477:string)  [unwired: 1 in]
        n297 = Equal?(x=w477, y=w478) -> (x = y?=w475:bool)
        n298 = case shown="True" w475 {
          frame False {
          }
          frame True {
            n299 = for {
              N: 4 -> [_]
              i -> [w481]
              n300 = Wait Until Next ms Multiple(millisecond multiple=u32 1000) -> ()  [unwired: 1 out]
              n301 = local write "Ring 1"(w481) -> ()
            }
          }
        }
      }
    }
    n302 = case shown="True" w455 {
      tunnel: w453 -> [_ w468]
      frame False {
      }
      frame True {
        n303 = local read "hour"() -> (w469:i32)
        n304 = Number To Decimal String(number=w468) -> (decimal integer string=w471:string)  [unwired: 1 in]
        n305 = Number To Decimal String(number=w469) -> (decimal integer string=w470:string)  [unwired: 1 in]
        n306 = Equal?(x=w470, y=w471) -> (x = y?=w467:bool)
        n307 = case shown="True" w467 {
          frame False {
          }
          frame True {
            n308 = for {
              N: 4 -> [_]
              i -> [w473]
              n309 = Wait Until Next ms Multiple(millisecond multiple=u32 1000) -> ()  [unwired: 1 out]
              n310 = local write "Ring 2"(w473) -> ()
            }
          }
        }
      }
    }
    n311 = case shown="True" w454 {
      tunnel: w453 -> [_ w463]
      frame False {
      }
      frame True {
        n312 = local read "hour"() -> (w460:i32)
        n313 = Number To Decimal String(number=w463) -> (decimal integer string=w462:string)  [unwired: 1 in]
        n314 = Number To Decimal String(number=w460) -> (decimal integer string=w461:string)  [unwired: 1 in]
        n315 = Equal?(x=w461, y=w462) -> (x = y?=w459:bool)
        n316 = case shown="True" w459 {
          frame False {
          }
          frame True {
            n317 = for {
              N: 4 -> [_]
              i -> [w465]
              n318 = Wait Until Next ms Multiple(millisecond multiple=u32 1000) -> ()  [unwired: 1 out]
              n319 = local write "Ring 3"(w465) -> ()
            }
          }
        }
      }
    }
    "For loop count - hour" <- w453
  }
  n320 = while {
    stop <- FALSE stop-if-true
    n321 = local read "Numeric 2"() -> (w494:i32)
    n322 = local read "Numeric 3"() -> (w486:i32)
    n323 = local read "Numeric"() -> (w497:i32)
    n324 = local read "temperature level 3"() -> (w485:bool)
    n325 = local read "temperature level 2"() -> (w492:bool)
    n326 = local read "check for level"() -> (w496:bool)
    n327 = local read "check for level 2"() -> (w490:bool)
    n328 = local read "check for level 3"() -> (w483:bool)
    n329 = local read "temperature level"() -> (w500:bool)
    n330 = Greater Or Equal?(x="Slide 3", y=w486) -> (x >= y?=w487:bool)
    n331 = Greater Or Equal?(x="Slide 2", y=w494) -> (x >= y?=w491:bool)
    n332 = Greater Or Equal?(x="Slide", y=w497) -> (x >= y?=w501:bool)
    n333 = And(x=w485, y=w487) -> (x .and. y?=w484:bool)
    n334 = And(x=w492, y=w491) -> (x .and. y?=w489:bool)
    n335 = And(x=w500, y=w501) -> (x .and. y?=w495:bool)
    n336 = case shown="False" w496 {
      tunnel: w495 -> [w508 _]
      frame False {
        n337 = case shown="False" w508 {
          frame False {
            n338 = local write "Ring 4"(u16 0 ("Ring 4")) -> ()
          }
          frame True {
            n339 = local write "Ring 4"(u16 4 ("Ring 4")) -> ()
          }
        }
      }
      frame True {
      }
    }
    n340 = case shown="False" w490 {
      tunnel: w489 -> [w505 _]
      frame False {
        n341 = case shown="True" w505 {
          frame False {
            n342 = local write "Ring 5"(u16 0 ("Ring 4")) -> ()
          }
          frame True {
            n343 = local write "Ring 5"(u16 4 ("Ring 4")) -> ()
          }
        }
      }
      frame True {
      }
    }
    n344 = case shown="False" w483 {
      tunnel: w484 -> [w502 _]
      frame False {
        n345 = case shown="False" w502 {
          frame False {
            n346 = local write "Ring 6"(u16 0 ("Ring 4")) -> ()
          }
          frame True {
            n347 = local write "Ring 6"(u16 4 ("Ring 4")) -> ()
          }
        }
      }
      frame True {
      }
    }
  }
  n348 = TCP Close Connection(connection ID=w11, error in (no error)=w10) -> (error out=w6:errorcluster)  [unwired: 1 in, 1 out]
  n349 = call <vilib>:"Clear Errors.vi"("error in (no error)"=w6) -> ()  [unwired: 6 in, 1 out]
